vi "CreateScriptingVI.vi"(8 "error in":errorcluster) -> (0 "error out":errorcluster)   [LabVIEW 2020, in "G-AI tests.lvlib"]
doc: "Creates a new VI that has a \"New VI\" function followed by a propertynode iwth different properties set to read/write. Also checks if the available properties are found. Used to test propertynode capabilities."
uses:
  G-AI tests.lvlib
  <vilib>/addons/_JKI Toolkits/Caraya/classes/Assert/Assert.lvclass
  <vilib>/addons/_JKI Toolkits/Caraya/classes/Test/Test.lvclass
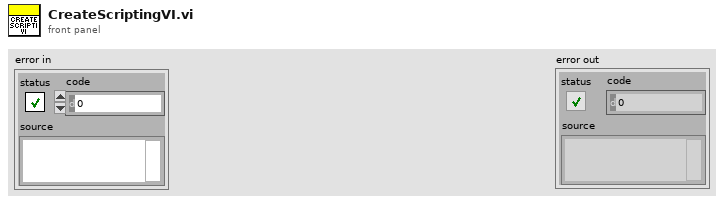
[diagram p1: front panel]
types:
  T1 = typedef "ASPM_ArrayOfUniqueIDStringDatanameShortnameLongname.ctl" = T2[]
  T2 = typedef "ASPM_UniqueIDStringDatanameShortnameLongname.ctl" = cluster{"Unique ID string":string, "Data name":string, "Short name (localized)":string, "Long name (localized)":string}
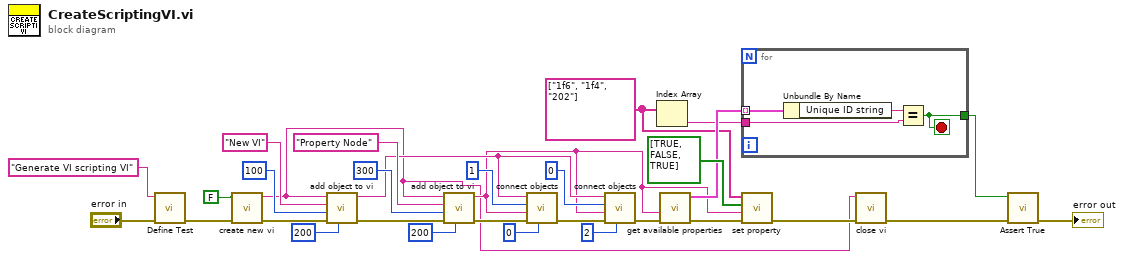
[diagram p0: block diagram]
diagram:
  w11 = string[] ["1f6", "1f4", "202"] ("property_ids")
  n1 = call <vilib>:"Define Test.vi"("error in (no error)"="error in", "Label (VI Title)"="Generate VI scripting VI") -> ("error out"=w7:errorcluster)  [unwired: 8 in, 1 out]
  n2 = call "create new vi.vi"("error in"=w7, "Show VI"=FALSE) -> ("error out"=w21:errorcluster, "vi id"=w2:string)  [unwired: 8 in]
  n3 = call "add object to vi.vi"("position_y"=i16 200, "error in (no error)"=w21, "position_x"=i16 100, "object_name"="New VI", "vi id"=w2) -> ("error out"=w22:errorcluster, "ctl id"=w25:string)  [unwired: 5 in]
  n4 = call "add object to vi.vi"("position_y"=i16 200, "error in (no error)"=w22, "position_x"=i16 300, "object_name"="Property Node", "vi id"=w2) -> ("error out"=w17:errorcluster, "ctl id"=w3:string)  [unwired: 5 in]
  n5 = call "connect objects.vi"("to object terminal index"=0, "error in"=w17, "to object id"=w3, "from object terminal index"=1, "from object id"=w25) -> ("error out"=w18:errorcluster)  [unwired: 6 in]
  n6 = call "connect objects.vi"("to object terminal index"=2, "error in"=w18, "to object id"=w3, "from object terminal index"=0, "from object id"=w25) -> ("error out"=w16:errorcluster)  [unwired: 6 in]
  n7 = Index Array(array=w11) -> (element=w10:string)  [unwired: 1 in]
  n8 = call "get available properties.vi"("error in"=w16, "propertynode_id"=w3) -> ("error out"=w15:errorcluster, "All Supported Properties"=w12:T1)  [unwired: 8 in]
  n9 = for {
    tunnel: w12 -> [w35] mode=indexing
    tunnel: w10 -> [w33]
    tunnel: [w32] -> w8
    stop <- w32 stop-if-true
    n10 = Unbundle By Name(w35) -> ("Unique ID string"=w34:string)
    n11 = Equal?(x=w34, y=w33) -> (x = y?=w32:bool)
  }
  n12 = call "set property.vi"("error in"=w15, "propertynode_id"=w3, "properties_iswrite"=bool[] [TRUE, FALSE, TRUE], "property_ids"=w11) -> ("error out"=w5:errorcluster)  [unwired: 7 in]
  n13 = call "close vi.vi"("error in"=w5, "vi id"=w2) -> ("error out"=w4:errorcluster)  [unwired: 9 in]
  n14 = call <vilib>:"Assert True.vi"("error in (no error)"=w4, "True?"=w8) -> ("error out"=→"error out":errorcluster)  [unwired: 8 in, 1 out]
